vi "水样测试.vi"(11 "数据标记表":string(combo)="N") -> ()   [LabVIEW 2016, in "斯坦道多参数.lvlib"]
panel:
  out "运行状态":u16(ring) items=["空闲", "水样测试", "标样核查"]
  out "多参数运行日志":string
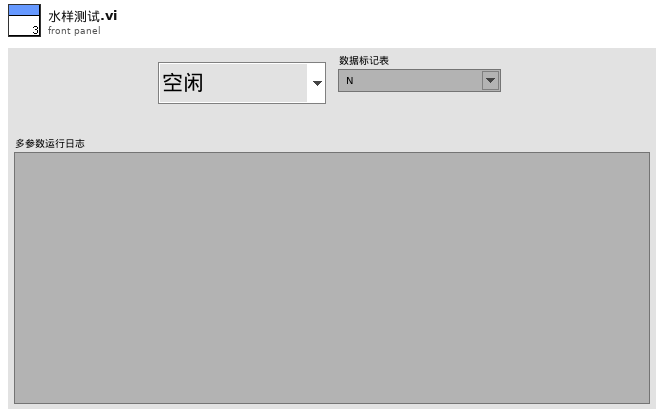
[diagram p1: front panel]
types:
  T1 = cluster{"水温":bool, "pH":bool, "DO":bool, "DOper":bool, "电导率":bool, "ORP":bool, "浊度":bool, "叶绿素a":bool, "藻密度":bool}
  T2 = cluster{"水样数据时间":timestamp, "检测值":cluster{"水温":dbl, "pH":dbl, "DO":dbl, "DOper":dbl, "电导率":dbl, "ORP":dbl, "浊度":dbl, "叶绿素a":dbl, "藻密度":dbl}}
  T3 = cluster{"水样数据时间":timestamp, "水样实测值":sgl, "单位":string, "水样数据标识":string, "信号值":sgl, "标样参考值":sgl, "因子编码":string, "探头温度":sgl}
  T4 = cluster{"ph":bool, "DO":bool, "Cond":bool, "Turb":bool, "叶绿素a":bool, "藻密度":bool, "ORP":bool}
  T5 = cluster{"CH":u16, "监测值":dbl, "温度偏移修正值":sgl, "信号值":sgl}
  T6 = cluster{"温度测量值":sgl, "测量值":sgl, "温度偏移修正值":sgl, "信号值":sgl}
  T7 = cluster{"温度测量值":sgl, "DO%":sgl, "DOmg/L":sgl, "温度偏移修正值":sgl}
  T8 = cluster{"测量量程":dbl, "测量精度":dbl, "测量间隔":dbl, "消解温度":dbl, "消解时长":dbl, "空白校准时间":timestamp, "曲线截距":dbl, "曲线斜率":dbl, "测量检出限":dbl, "测量信号值":dbl, "线性相关系数":dbl, "二次多项式系数":dbl, "标样校准时间":timestamp, "稀释倍数":dbl, "三项式系数":dbl, "空白标定系数":dbl, "量程系数":dbl, "F0/ORPA":dbl, "F1/ORPB":dbl, "F2/ORPK":dbl, "F3":dbl, "F4":dbl, "F5":dbl, "F6":dbl, "F7":dbl, "X0/滴定数":dbl, "量程":dbl}
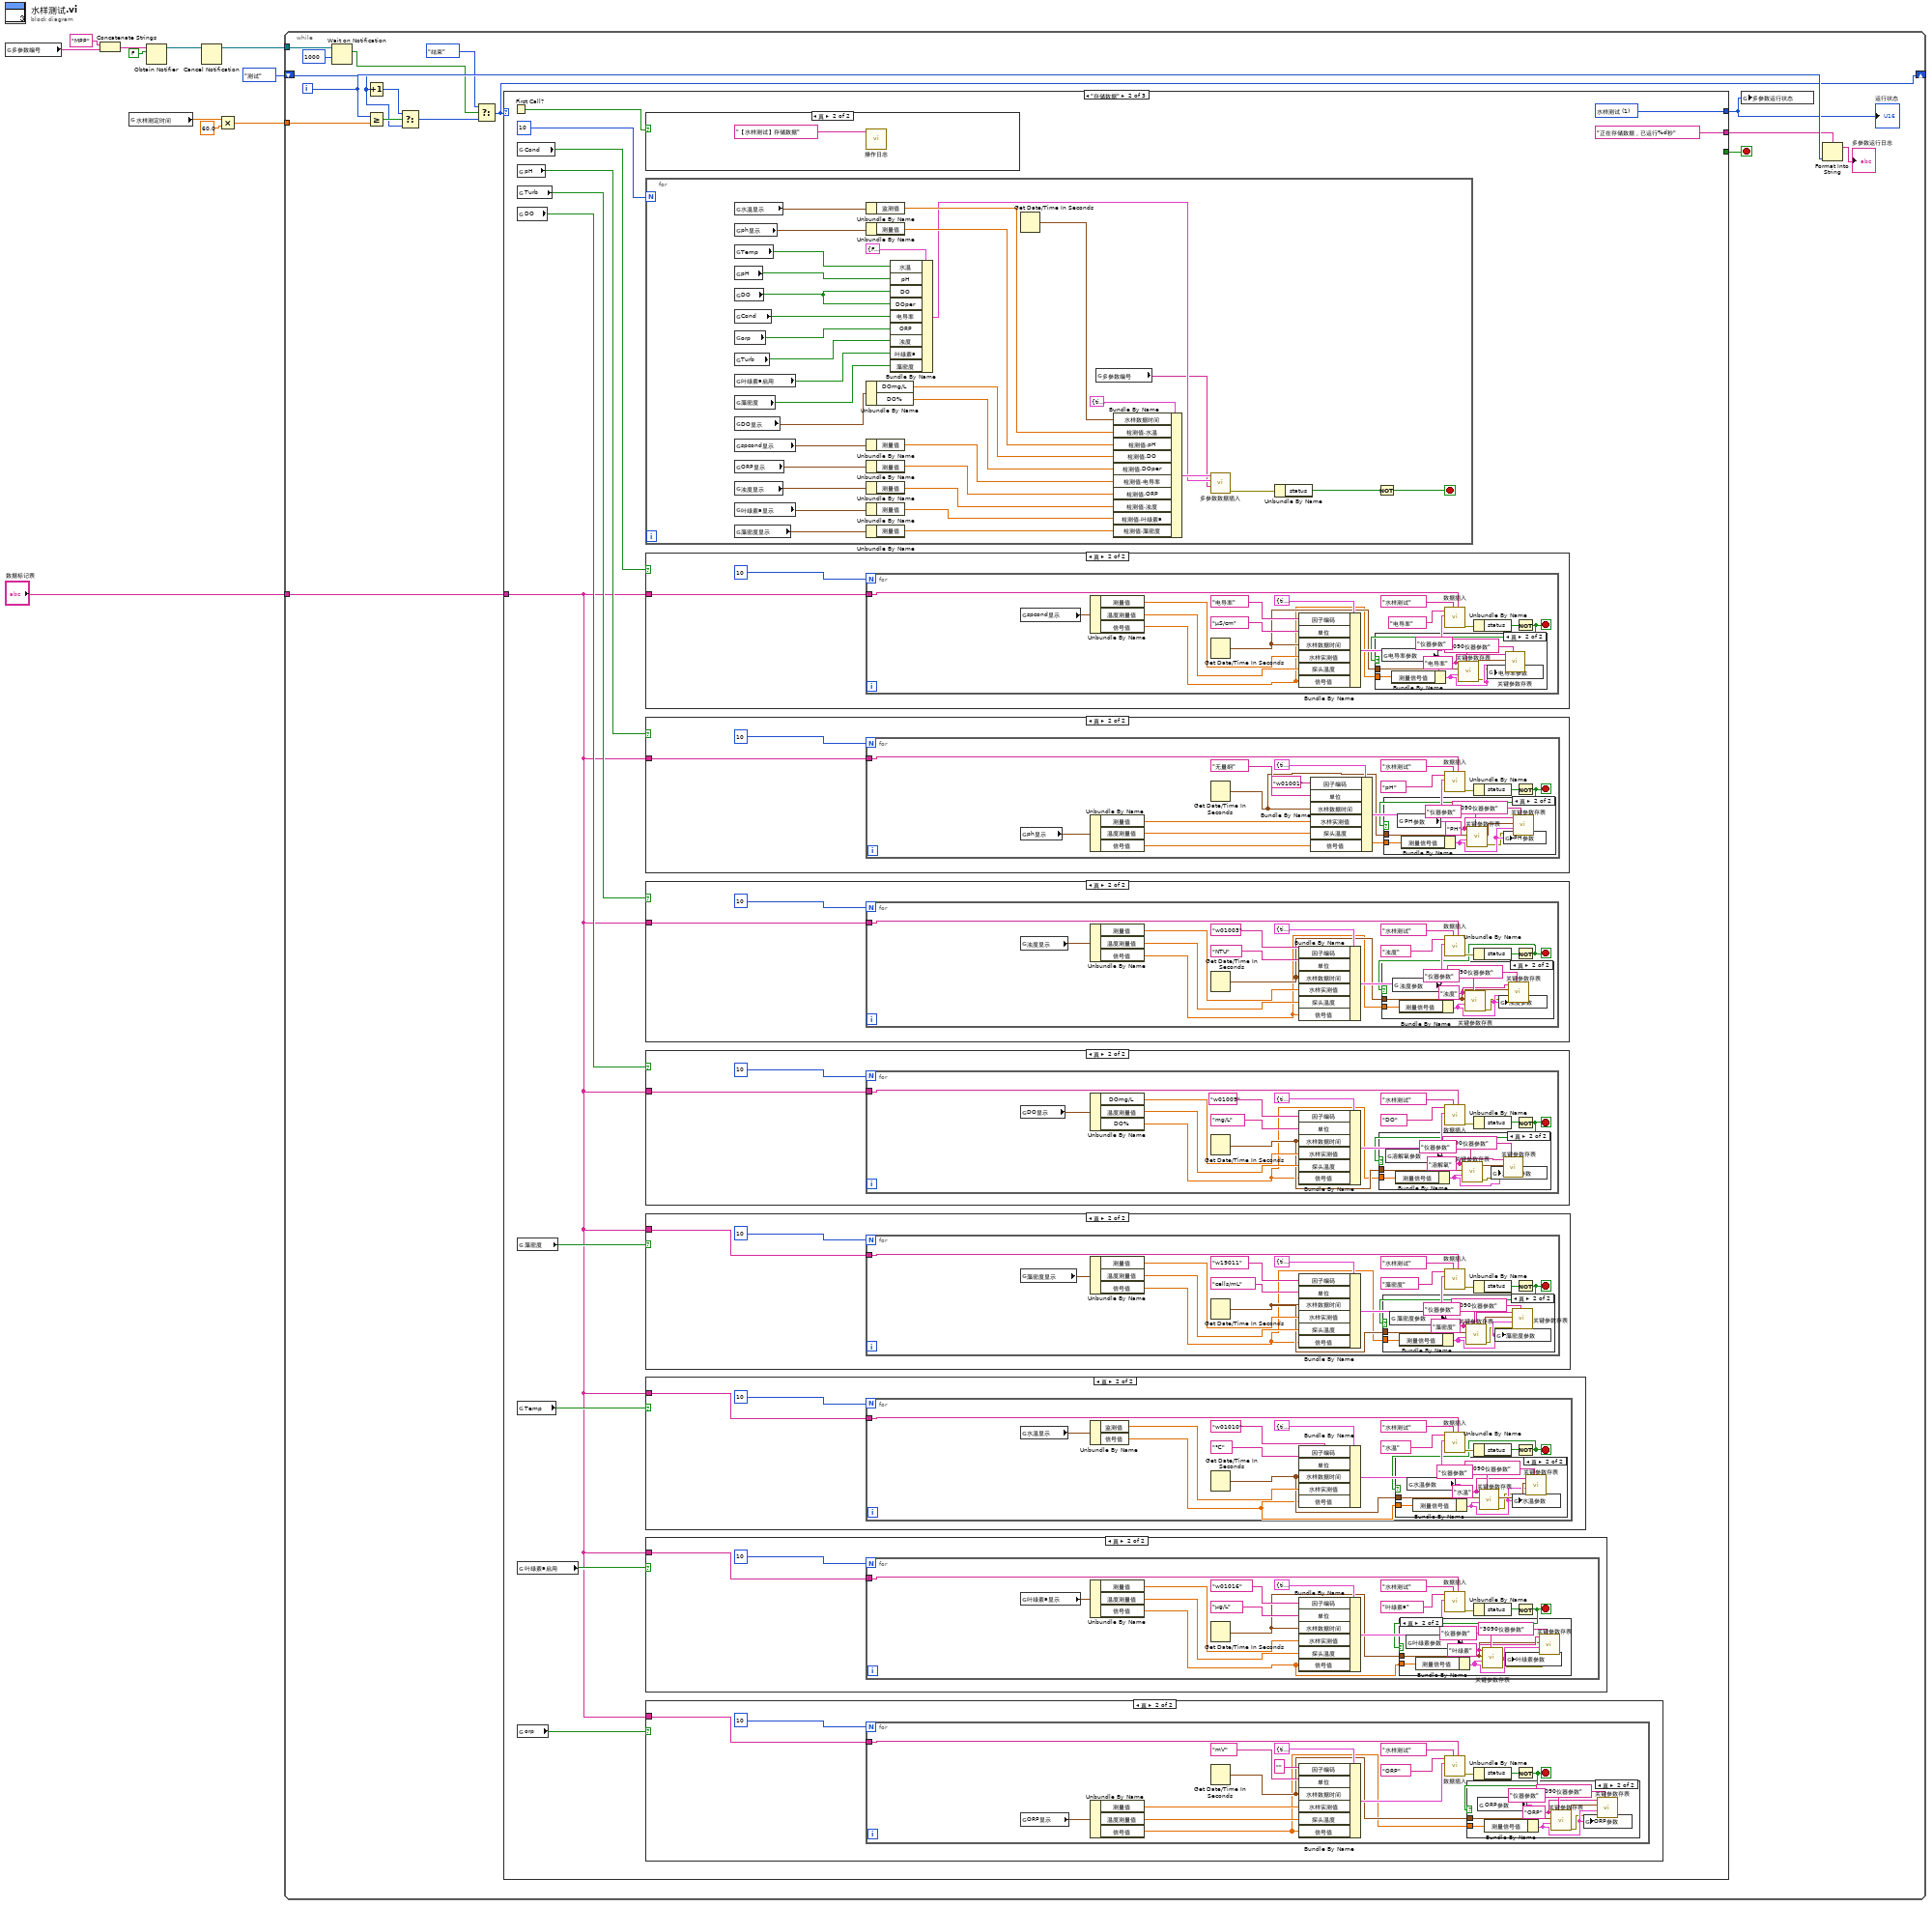
[diagram p0: block diagram]
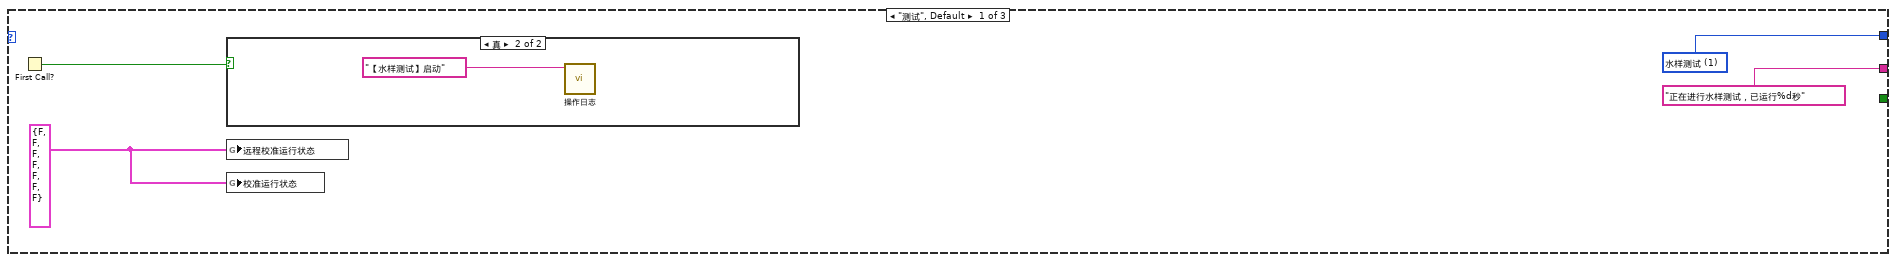
[diagram p2: hidden frame]
diagram:
  n1 = global read "多参数全局变量.vi" "多参数编号"() -> (w2:string)
  n2 = Concatenate Strings("MPP" ("名称（未命名）"), w2) -> (w3:string)
  n3 = global read "断电保存变量.vi" "水样测定时间"() -> (w1:dbl)
  n4 = Obtain Notifier(name (unnamed)=w3, notification data type=FALSE) -> (notifier out=w6:refnum<notifier>)  [unwired: 2 in, 2 out]
  n5 = Cancel Notification(0:w6) -> (8:w5:refnum<notifier>)  [unwired: 1 in, 2 out]
  n6 = Multiply(x=w1, y=60.0) -> (x*y=w10:dbl)
  n7 = while {
    tunnel: w10 -> [w27]
    shift-right: [w14] -> _
    shift-left: enum16{"测试", "存储数据", "结束"}."测试" ("枚举") -> [w21]
    tunnel: w5 -> [w19]
    tunnel: "数据标记表" -> [w13]
    i -> [w25]
    stop <- w26 stop-if-true
    n8 = Wait on Notification(notifier=w19, timeout in ms (-1)=1000 ("超时毫秒(-1)")) -> (notification=w17:bool)  [unwired: 2 in, 3 out]
    n9 = Increment(x=w21) -> (x+1=w20:enum16{"测试", "存储数据", "结束"})
    n10 = Greater Or Equal?(x=w25, y=w27) -> (x >= y?=w22:bool)
    n11 = Select(t=w20, s=w22, f=w21) -> (s? t:f=w15:enum16{"测试", "存储数据", "结束"})
    n12 = Select(t=enum16{"测试", "存储数据", "结束"}."结束" ("枚举"), s=w17, f=w15) -> (s? t:f=w14:enum16{"测试", "存储数据", "结束"})
    n13 = case shown="\"存储数据\"" w14 {
      tunnel: [_ _ TRUE] -> w26
      tunnel: ["正在进行水样测试，已运行%d秒" ("格式字符串") "正在存储数据，已运行%d秒" ("格式字符串") "测试停止，累计运行%d秒" ("格式字符串")] -> w24
      tunnel: [w30 w38 w281] -> w12
      tunnel: w13 -> [_ w35 _]
      frame "测试", Default {
        w28 = T4 {"ph"=FALSE, "DO"=FALSE, "Cond"=FALSE, "Turb"=FALSE, "叶绿素a"=FALSE, "藻密度"=FALSE, "ORP"=FALSE} ("校准运行状态")
        w30 = u16 1 items=["空闲", "水样测试", "标样核查"] ("多参数运行状态")
        n14 = First Call?() -> (First Call?: T/F=w29:bool)
        n15 = case shown="真" w29 {
          frame False {
          }
          frame True {
            n16 = call "操作日志.vi"("日志信息"="【水样测试】启动") -> ()  [unwired: 10 in, 1 out]
          }
        }
        n17 = global write "多参数全局变量.vi" "远程校准运行状态"(w28) -> ()
        n18 = global write "多参数全局变量.vi" "校准运行状态"(w28) -> ()
      }
      frame "存储数据" {
        w38 = u16 1 items=["空闲", "水样测试", "标样核查"] ("多参数运行状态")
        n19 = First Call?() -> (First Call?: T/F=w36:bool)
        n20 = global read "断电保存变量.vi" "Cond"() -> (w43:bool)
        n21 = global read "断电保存变量.vi" "pH"() -> (w41:bool)
        n22 = global read "断电保存变量.vi" "Turb"() -> (w44:bool)
        n23 = global read "断电保存变量.vi" "DO"() -> (w42:bool)
        n24 = global read "断电保存变量.vi" "藻密度"() -> (w37:bool)
        n25 = global read "断电保存变量.vi" "Temp"() -> (w40:bool)
        n26 = global read "断电保存变量.vi" "叶绿素a启用"() -> (w45:bool)
        n27 = global read "断电保存变量.vi" "orp"() -> (w34:bool)
        n28 = case shown="真" w36 {
          frame False {
          }
          frame True {
            n29 = call "操作日志.vi"("日志信息"="【水样测试】存储数据") -> ()  [unwired: 10 in, 1 out]
          }
        }
        n30 = for {
          N: 10 -> [_]
          stop <- w47 stop-if-true
          n31 = global read "多参数全局变量.vi" "水温显示"() -> (w76:T5)
          n32 = global read "多参数全局变量.vi" "ph显示"() -> (w74:T6)
          n33 = global read "断电保存变量.vi" "Temp"() -> (w54:bool)
          n34 = global read "断电保存变量.vi" "pH"() -> (w58:bool)
          n35 = global read "断电保存变量.vi" "DO"() -> (w50:bool)
          n36 = global read "断电保存变量.vi" "Cond"() -> (w57:bool)
          n37 = global read "断电保存变量.vi" "orp"() -> (w53:bool)
          n38 = global read "断电保存变量.vi" "Turb"() -> (w56:bool)
          n39 = global read "断电保存变量.vi" "叶绿素a启用"() -> (w52:bool)
          n40 = global read "断电保存变量.vi" "藻密度"() -> (w55:bool)
          n41 = global read "多参数全局变量.vi" "DO显示"() -> (w72:T7)
          n42 = global read "多参数全局变量.vi" "spcond显示"() -> (w69:T6)
          n43 = global read "多参数全局变量.vi" "ORP显示"() -> (w67:T6)
          n44 = global read "多参数全局变量.vi" "浊度显示"() -> (w65:T6)
          n45 = global read "多参数全局变量.vi" "叶绿素a显示"() -> (w61:T6)
          n46 = global read "多参数全局变量.vi" "藻密度显示"() -> (w63:T6)
          n47 = Unbundle By Name(w76) -> ("监测值"=w75:dbl)
          n48 = Unbundle By Name(w74) -> ("测量值"=w73:sgl)
          n49 = Unbundle By Name(w72) -> ("DOmg/L"=w71:sgl, "DO%"=w70:sgl)
          n50 = Unbundle By Name(w69) -> ("测量值"=w68:sgl)
          n51 = Unbundle By Name(w67) -> ("测量值"=w66:sgl)
          n52 = Unbundle By Name(w65) -> ("测量值"=w64:sgl)
          n53 = Unbundle By Name(w61) -> ("测量值"=w60:sgl)
          n54 = Unbundle By Name(w63) -> ("测量值"=w62:sgl)
          n55 = Bundle By Name(cluster=T1 {"水温"=FALSE, "pH"=FALSE, "DO"=FALSE, "DOper"=FALSE, "电导率"=FALSE, "ORP"=FALSE, "浊度"=FALSE, "叶绿素a"=FALSE, "藻密度"=FALSE} ("columns enable"), "水温"=w54, "pH"=w58, "DO"=w50, "DOper"=w50, "电导率"=w57, "ORP"=w53, "浊度"=w56, "叶绿素a"=w52, "藻密度"=w55) -> (w51:T1)
          n56 = Get Date/Time In Seconds() -> (seconds since 1Jan1904=w77:timestamp)
          n57 = global read "多参数全局变量.vi" "多参数编号"() -> (w46:string)
          n58 = Bundle By Name(cluster=T2 {"水样数据时间"=timestamp(0 s since 1904-01-01), "检测值"={"水温"=0.0, "pH"=0.0, "DO"=0.0, "DOper"=0.0, "电导率"=0.0, "ORP"=0.0, "浊度"=0.0, "叶绿素a"=0.0, "藻密度"=0.0}} ("data in"), "水样数据时间"=w77, "检测值.水温"=w75, "检测值.pH"=w73, "检测值.DO"=w71, "检测值.DOper"=w70, "检测值.电导率"=w68, "检测值.ORP"=w66, "检测值.浊度"=w64, "检测值.叶绿素a"=w60, "检测值.藻密度"=w62) -> (w78:T2)
          n59 = call "多参数数据插入.vi"("编号"=w46, "columns enable"=w51, "data in"=w78) -> ("error out"=w49:errorcluster)  [unwired: 8 in]
          n60 = Unbundle By Name(w49) -> ("status"=w48:bool)
          n61 = Not(x=w48) -> (.not. x?=w47:bool)
        }
        n62 = case shown="真" w43 {
          tunnel: w35 -> [_ w182]
          frame False {
          }
          frame True {
            n63 = for {
              N: 10 -> [_]
              tunnel: w182 -> [w193]
              stop <- w185 stop-if-true
              n64 = global read "多参数全局变量.vi" "spcond显示"() -> (w192:T6)
              n65 = Unbundle By Name(w192) -> ("测量值"=w191:sgl, "温度测量值"=w190:sgl, "信号值"=w183:sgl)
              n66 = Get Date/Time In Seconds() -> (seconds since 1Jan1904=w184:timestamp)
              n67 = Bundle By Name(cluster=T3 {"水样数据时间"=timestamp(0 s since 1904-01-01), "水样实测值"=0.0, "单位"="", "水样数据标识"="N", "信号值"=0.0, "标样参考值"=0.0, "因子编码"="", "探头温度"=0.0} ("data in"), "因子编码"="电导率", "单位"="μS/cm", "水样数据时间"=w184, "水样实测值"=w191, "探头温度"=w190, "信号值"=w183) -> (w196:T3)
              n68 = call "数据插入.vi"("数据类型"=w193, "测量模式"="水样测试", "data in"=w196, "table输入"="电导率") -> ("error out"=w189:errorcluster)  [unwired: 7 in]
              n69 = Unbundle By Name(w189) -> ("status"=w188:bool)
              n70 = Not(x=w188) -> (.not. x?=w185:bool)
              n71 = case shown="真" w185 {
                tunnel: w184 -> [_ w200]
                tunnel: w183 -> [_ w204]
                frame False {
                }
                frame True {
                  w203 = "电导率" ("仪器名称")
                  n72 = global read "断电保存变量.vi" "电导率参数"() -> (w205:T8)
                  n73 = Bundle By Name(cluster=w205, "测量信号值"=w204) -> (w199:T8)
                  n74 = call "关键参数存表.vi"("table"="仪器参数", "仪器参数"=w199, "datatime"=w200, "仪器名称"=w203) -> ("error out"=w198:errorcluster)  [unwired: 7 in]
                  n75 = global write "断电保存变量.vi" "电导率参数"(w199) -> ()
                  n76 = call "关键参数存表.vi"("table"="3090仪器参数", "error in (no error)"=w198, "仪器参数"=w199, "datatime"=w200, "仪器名称"=w203) -> ()  [unwired: 6 in, 1 out]
                }
              }
            }
          }
        }
        n77 = case shown="真" w41 {
          tunnel: w35 -> [_ w232]
          frame False {
          }
          frame True {
            n78 = for {
              N: 10 -> [_]
              tunnel: w232 -> [w242]
              stop <- w235 stop-if-true
              n79 = global read "多参数全局变量.vi" "ph显示"() -> (w241:T6)
              n80 = Unbundle By Name(w241) -> ("测量值"=w240:sgl, "温度测量值"=w239:sgl, "信号值"=w233:sgl)
              n81 = Get Date/Time In Seconds() -> (seconds since 1Jan1904=w234:timestamp)
              n82 = Bundle By Name(cluster=T3 {"水样数据时间"=timestamp(0 s since 1904-01-01), "水样实测值"=0.0, "单位"="", "水样数据标识"="N", "信号值"=0.0, "标样参考值"=0.0, "因子编码"="", "探头温度"=0.0} ("data in"), "因子编码"="w01001", "单位"="无量纲", "水样数据时间"=w234, "水样实测值"=w240, "探头温度"=w239, "信号值"=w233) -> (w246:T3)
              n83 = call "数据插入.vi"("数据类型"=w242, "测量模式"="水样测试", "data in"=w246, "table输入"="pH") -> ("error out"=w238:errorcluster)  [unwired: 7 in]
              n84 = Unbundle By Name(w238) -> ("status"=w237:bool)
              n85 = Not(x=w237) -> (.not. x?=w235:bool)
              n86 = case shown="真" w235 {
                tunnel: w234 -> [_ w250]
                tunnel: w233 -> [_ w254]
                frame False {
                }
                frame True {
                  w253 = "PH" ("仪器名称")
                  n87 = global read "断电保存变量.vi" "PH参数"() -> (w255:T8)
                  n88 = Bundle By Name(cluster=w255, "测量信号值"=w254) -> (w249:T8)
                  n89 = call "关键参数存表.vi"("table"="仪器参数", "仪器参数"=w249, "datatime"=w250, "仪器名称"=w253) -> ("error out"=w248:errorcluster)  [unwired: 7 in]
                  n90 = global write "断电保存变量.vi" "PH参数"(w249) -> ()
                  n91 = call "关键参数存表.vi"("table"="3090仪器参数", "error in (no error)"=w248, "仪器参数"=w249, "datatime"=w250, "仪器名称"=w253) -> ()  [unwired: 6 in, 1 out]
                }
              }
            }
          }
        }
        n92 = case shown="真" w44 {
          tunnel: w35 -> [_ w157]
          frame False {
          }
          frame True {
            n93 = for {
              N: 10 -> [_]
              tunnel: w157 -> [w167]
              stop <- w160 stop-if-true
              n94 = global read "多参数全局变量.vi" "浊度显示"() -> (w166:T6)
              n95 = Unbundle By Name(w166) -> ("测量值"=w165:sgl, "温度测量值"=w164:sgl, "信号值"=w158:sgl)
              n96 = Get Date/Time In Seconds() -> (seconds since 1Jan1904=w159:timestamp)
              n97 = Bundle By Name(cluster=T3 {"水样数据时间"=timestamp(0 s since 1904-01-01), "水样实测值"=0.0, "单位"="", "水样数据标识"="N", "信号值"=0.0, "标样参考值"=0.0, "因子编码"="", "探头温度"=0.0} ("data in"), "因子编码"="w01003", "单位"="NTU", "水样数据时间"=w159, "水样实测值"=w165, "探头温度"=w164, "信号值"=w158) -> (w171:T3)
              n98 = call "数据插入.vi"("数据类型"=w167, "测量模式"="水样测试", "data in"=w171, "table输入"="浊度") -> ("error out"=w163:errorcluster)  [unwired: 7 in]
              n99 = Unbundle By Name(w163) -> ("status"=w162:bool)
              n100 = Not(x=w162) -> (.not. x?=w160:bool)
              n101 = case shown="真" w160 {
                tunnel: w159 -> [_ w175]
                tunnel: w158 -> [_ w179]
                frame False {
                }
                frame True {
                  w176 = "浊度" ("仪器名称")
                  n102 = global read "断电保存变量.vi" "浊度参数"() -> (w180:T8)
                  n103 = Bundle By Name(cluster=w180, "测量信号值"=w179) -> (w174:T8)
                  n104 = call "关键参数存表.vi"("table"="仪器参数", "仪器参数"=w174, "datatime"=w175, "仪器名称"=w176) -> ("error out"=w173:errorcluster)  [unwired: 7 in]
                  n105 = global write "断电保存变量.vi" "浊度参数"(w174) -> ()
                  n106 = call "关键参数存表.vi"("table"="3090仪器参数", "error in (no error)"=w173, "仪器参数"=w174, "datatime"=w175, "仪器名称"=w176) -> ()  [unwired: 6 in, 1 out]
                }
              }
            }
          }
        }
        n107 = case shown="真" w42 {
          tunnel: w35 -> [_ w207]
          frame False {
          }
          frame True {
            n108 = for {
              N: 10 -> [_]
              tunnel: w207 -> [w217]
              stop <- w210 stop-if-true
              n109 = global read "多参数全局变量.vi" "DO显示"() -> (w216:T7)
              n110 = Unbundle By Name(w216) -> ("DOmg/L"=w215:sgl, "温度测量值"=w214:sgl, "DO%"=w208:sgl)
              n111 = Get Date/Time In Seconds() -> (seconds since 1Jan1904=w209:timestamp)
              n112 = Bundle By Name(cluster=T3 {"水样数据时间"=timestamp(0 s since 1904-01-01), "水样实测值"=0.0, "单位"="", "水样数据标识"="N", "信号值"=0.0, "标样参考值"=0.0, "因子编码"="", "探头温度"=0.0} ("data in"), "因子编码"="w01009", "单位"="mg/L", "水样数据时间"=w209, "水样实测值"=w215, "探头温度"=w214, "信号值"=w208) -> (w221:T3)
              n113 = call "数据插入.vi"("数据类型"=w217, "测量模式"="水样测试", "data in"=w221, "table输入"="DO") -> ("error out"=w213:errorcluster)  [unwired: 7 in]
              n114 = Unbundle By Name(w213) -> ("status"=w212:bool)
              n115 = Not(x=w212) -> (.not. x?=w210:bool)
              n116 = case shown="真" w210 {
                tunnel: w209 -> [_ w227]
                tunnel: w208 -> [_ w229]
                frame False {
                }
                frame True {
                  w228 = "溶解氧" ("仪器名称")
                  n117 = global read "断电保存变量.vi" "溶解氧参数"() -> (w230:T8)
                  n118 = Bundle By Name(cluster=w230, "测量信号值"=w229) -> (w226:T8)
                  n119 = call "关键参数存表.vi"("table"="仪器参数", "仪器参数"=w226, "datatime"=w227, "仪器名称"=w228) -> ("error out"=w225:errorcluster)  [unwired: 7 in]
                  n120 = global write "断电保存变量.vi" "溶解氧参数"(w226) -> ()
                  n121 = call "关键参数存表.vi"("table"="3090仪器参数", "error in (no error)"=w225, "仪器参数"=w226, "datatime"=w227, "仪器名称"=w228) -> ()  [unwired: 6 in, 1 out]
                }
              }
            }
          }
        }
        n122 = case shown="真" w37 {
          tunnel: w35 -> [_ w107]
          frame False {
          }
          frame True {
            n123 = for {
              N: 10 -> [_]
              tunnel: w107 -> [w116]
              stop <- w108 stop-if-true
              n124 = global read "多参数全局变量.vi" "藻密度显示"() -> (w115:T6)
              n125 = Unbundle By Name(w115) -> ("测量值"=w121:sgl, "温度测量值"=w119:sgl, "信号值"=w109:sgl)
              n126 = Get Date/Time In Seconds() -> (seconds since 1Jan1904=w110:timestamp)
              n127 = Bundle By Name(cluster=T3 {"水样数据时间"=timestamp(0 s since 1904-01-01), "水样实测值"=0.0, "单位"="", "水样数据标识"="N", "信号值"=0.0, "标样参考值"=0.0, "因子编码"="", "探头温度"=0.0} ("data in"), "因子编码"="w19011", "单位"="cells/mL", "水样数据时间"=w110, "水样实测值"=w121, "探头温度"=w119, "信号值"=w109) -> (w111:T3)
              n128 = call "数据插入.vi"("数据类型"=w116, "测量模式"="水样测试", "data in"=w111, "table输入"="藻密度") -> ("error out"=w114:errorcluster)  [unwired: 7 in]
              n129 = Unbundle By Name(w114) -> ("status"=w113:bool)
              n130 = Not(x=w113) -> (.not. x?=w108:bool)
              n131 = case shown="真" w108 {
                tunnel: w110 -> [_ w126]
                tunnel: w109 -> [_ w129]
                frame False {
                }
                frame True {
                  w127 = "藻密度" ("仪器名称")
                  n132 = global read "断电保存变量.vi" "藻密度参数"() -> (w130:T8)
                  n133 = Bundle By Name(cluster=w130, "测量信号值"=w129) -> (w125:T8)
                  n134 = call "关键参数存表.vi"("table"="仪器参数", "仪器参数"=w125, "datatime"=w126, "仪器名称"=w127) -> ("error out"=w124:errorcluster)  [unwired: 7 in]
                  n135 = global write "断电保存变量.vi" "藻密度参数"(w125) -> ()
                  n136 = call "关键参数存表.vi"("table"="3090仪器参数", "error in (no error)"=w124, "仪器参数"=w125, "datatime"=w126, "仪器名称"=w127) -> ()  [unwired: 6 in, 1 out]
                }
              }
            }
          }
        }
        n137 = case shown="真" w40 {
          tunnel: w35 -> [_ w257]
          frame False {
          }
          frame True {
            n138 = for {
              N: 10 -> [_]
              tunnel: w257 -> [w266]
              stop <- w260 stop-if-true
              n139 = global read "多参数全局变量.vi" "水温显示"() -> (w265:T5)
              n140 = Unbundle By Name(w265) -> ("监测值"=w264:dbl, "信号值"=w258:sgl)
              n141 = Get Date/Time In Seconds() -> (seconds since 1Jan1904=w259:timestamp)
              n142 = Bundle By Name(cluster=T3 {"水样数据时间"=timestamp(0 s since 1904-01-01), "水样实测值"=0.0, "单位"="", "水样数据标识"="N", "信号值"=0.0, "标样参考值"=0.0, "因子编码"="", "探头温度"=0.0} ("data in"), "因子编码"="w01010", "单位"="℃", "水样数据时间"=w259, "水样实测值"=w264, "信号值"=w258) -> (w270:T3)
              n143 = call "数据插入.vi"("数据类型"=w266, "测量模式"="水样测试", "data in"=w270, "table输入"="水温") -> ("error out"=w263:errorcluster)  [unwired: 7 in]
              n144 = Unbundle By Name(w263) -> ("status"=w262:bool)
              n145 = Not(x=w262) -> (.not. x?=w260:bool)
              n146 = case shown="真" w260 {
                tunnel: w259 -> [_ w275]
                tunnel: w258 -> [_ w278]
                frame False {
                }
                frame True {
                  w276 = "水温" ("仪器名称")
                  n147 = global read "断电保存变量.vi" "水温参数"() -> (w279:T8)
                  n148 = Bundle By Name(cluster=w279, "测量信号值"=w278) -> (w274:T8)
                  n149 = call "关键参数存表.vi"("table"="仪器参数", "仪器参数"=w274, "datatime"=w275, "仪器名称"=w276) -> ("error out"=w273:errorcluster)  [unwired: 7 in]
                  n150 = global write "断电保存变量.vi" "水温参数"(w274) -> ()
                  n151 = call "关键参数存表.vi"("table"="3090仪器参数", "error in (no error)"=w273, "仪器参数"=w274, "datatime"=w275, "仪器名称"=w276) -> ()  [unwired: 6 in, 1 out]
                }
              }
            }
          }
        }
        n152 = case shown="真" w45 {
          tunnel: w35 -> [_ w132]
          frame False {
          }
          frame True {
            n153 = for {
              N: 10 -> [_]
              tunnel: w132 -> [w141]
              stop <- w135 stop-if-true
              n154 = global read "多参数全局变量.vi" "叶绿素a显示"() -> (w140:T6)
              n155 = Unbundle By Name(w140) -> ("测量值"=w146:sgl, "温度测量值"=w145:sgl, "信号值"=w134:sgl)
              n156 = Get Date/Time In Seconds() -> (seconds since 1Jan1904=w133:timestamp)
              n157 = Bundle By Name(cluster=T3 {"水样数据时间"=timestamp(0 s since 1904-01-01), "水样实测值"=0.0, "单位"="", "水样数据标识"="N", "信号值"=0.0, "标样参考值"=0.0, "因子编码"="", "探头温度"=0.0} ("data in"), "因子编码"="w01016", "单位"="μg/L", "水样数据时间"=w133, "水样实测值"=w146, "探头温度"=w145, "信号值"=w134) -> (w143:T3)
              n158 = call "数据插入.vi"("数据类型"=w141, "测量模式"="水样测试", "data in"=w143, "table输入"="叶绿素a") -> ("error out"=w139:errorcluster)  [unwired: 7 in]
              n159 = Unbundle By Name(w139) -> ("status"=w138:bool)
              n160 = Not(x=w138) -> (.not. x?=w135:bool)
              n161 = case shown="真" w135 {
                tunnel: w133 -> [_ w150]
                tunnel: w134 -> [_ w154]
                frame False {
                }
                frame True {
                  w151 = "叶绿素" ("仪器名称")
                  n162 = global read "断电保存变量.vi" "叶绿素参数"() -> (w155:T8)
                  n163 = Bundle By Name(cluster=w155, "测量信号值"=w154) -> (w149:T8)
                  n164 = call "关键参数存表.vi"("table"="仪器参数", "仪器参数"=w149, "datatime"=w150, "仪器名称"=w151) -> ("error out"=w148:errorcluster)  [unwired: 7 in]
                  n165 = global write "断电保存变量.vi" "叶绿素参数"(w149) -> ()
                  n166 = call "关键参数存表.vi"("table"="3090仪器参数", "error in (no error)"=w148, "仪器参数"=w149, "datatime"=w150, "仪器名称"=w151) -> ()  [unwired: 6 in, 1 out]
                }
              }
            }
          }
        }
        n167 = case shown="真" w34 {
          tunnel: w35 -> [_ w81]
          frame False {
          }
          frame True {
            n168 = for {
              N: 10 -> [_]
              tunnel: w81 -> [w90]
              stop <- w84 stop-if-true
              n169 = global read "多参数全局变量.vi" "ORP显示"() -> (w89:T6)
              n170 = Unbundle By Name(w89) -> ("测量值"=w95:sgl, "温度测量值"=w93:sgl, "信号值"=w82:sgl)
              n171 = Get Date/Time In Seconds() -> (seconds since 1Jan1904=w83:timestamp)
              n172 = Bundle By Name(cluster=T3 {"水样数据时间"=timestamp(0 s since 1904-01-01), "水样实测值"=0.0, "单位"="", "水样数据标识"="N", "信号值"=0.0, "标样参考值"=0.0, "因子编码"="", "探头温度"=0.0} ("data in"), "因子编码"="", "单位"="mV", "水样数据时间"=w83, "水样实测值"=w95, "探头温度"=w93, "信号值"=w82) -> (w91:T3)
              n173 = call "数据插入.vi"("数据类型"=w90, "测量模式"="水样测试", "data in"=w91, "table输入"="ORP") -> ("error out"=w88:errorcluster)  [unwired: 7 in]
              n174 = Unbundle By Name(w88) -> ("status"=w87:bool)
              n175 = Not(x=w87) -> (.not. x?=w84:bool)
              n176 = case shown="真" w84 {
                tunnel: w83 -> [_ w100]
                tunnel: w82 -> [_ w103]
                frame False {
                }
                frame True {
                  w101 = "ORP" ("仪器名称")
                  n177 = global read "断电保存变量.vi" "ORP参数"() -> (w104:T8)
                  n178 = Bundle By Name(cluster=w104, "测量信号值"=w103) -> (w99:T8)
                  n179 = call "关键参数存表.vi"("table"="仪器参数", "仪器参数"=w99, "datatime"=w100, "仪器名称"=w101) -> ("error out"=w98:errorcluster)  [unwired: 7 in]
                  n180 = global write "断电保存变量.vi" "ORP参数"(w99) -> ()
                  n181 = call "关键参数存表.vi"("table"="3090仪器参数", "error in (no error)"=w98, "仪器参数"=w99, "datatime"=w100, "仪器名称"=w101) -> ()  [unwired: 6 in, 1 out]
                }
              }
            }
          }
        }
      }
      frame "结束" {
        w281 = u16 0 items=["空闲", "水样测试", "标样核查"] ("多参数运行状态")
        n182 = First Call?() -> (First Call?: T/F=w280:bool)
        n183 = case shown="真" w280 {
          frame False {
          }
          frame True {
            n184 = call "操作日志.vi"("日志信息"="【水样测试】结束") -> ()  [unwired: 10 in, 1 out]
          }
        }
      }
    }
    "运行状态" <- w12
    n185 = global write "多参数全局变量.vi" "多参数运行状态"(w12) -> ()
    n186 = Format Into String(format string=w24, w25) -> (resulting string=→"多参数运行日志":string)  [unwired: 2 in, 1 out]
  }
